vi "Read Channels Enqueuers.vi"(8 "error in (no error)":errorcluster, 11 "Sequencer in":refnum<class "Sequencer.lvclass">) -> (0 "error out":errorcluster, 2 "Channels Enqueuers":refnum<class "Message Enqueuer.lvclass">[](array[class]), 3 "Sequencer out":refnum<class "Sequencer.lvclass">)   [LabVIEW 2015, in "Sequencer.lvlib" / "Sequencer.lvclass"]
uses:
  Sequencer.lvclass
  <vilib>/ActorFramework/Message Enqueuer/Message Enqueuer.lvclass
  Sequencer.lvclass/Sequencer.ctl
  SequencerConfig.lvclass
  SequencerInfo.lvclass
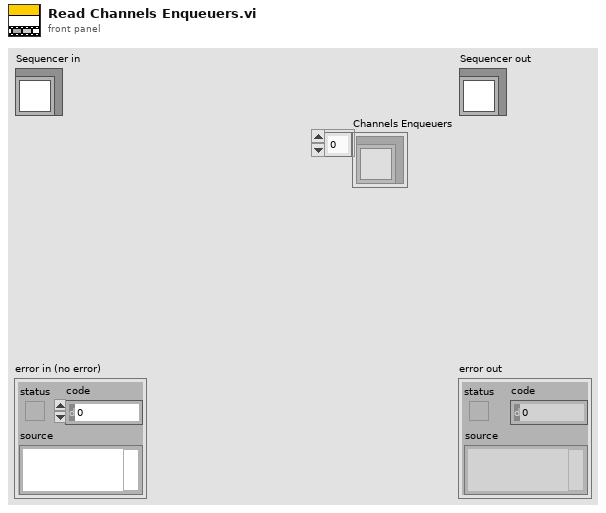
[diagram p1: front panel]
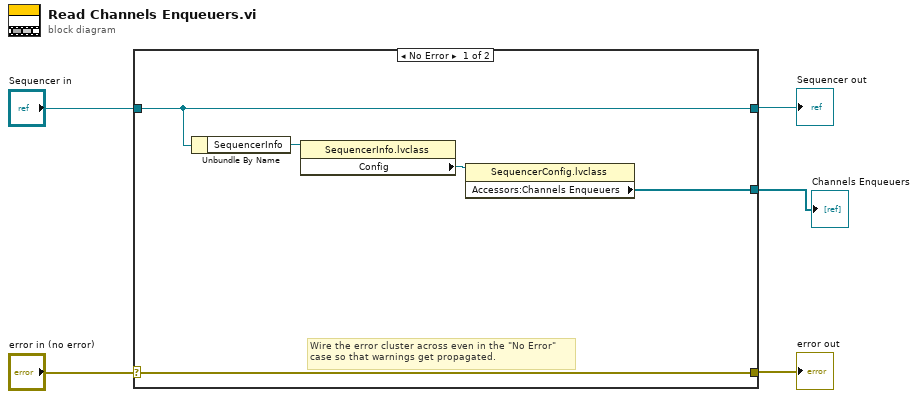
[diagram p0: block diagram]
diagram:
  n1 = case shown="No Error" "error in (no error)" {
    selector: "error in (no error)" -> [w10 w12]
    tunnel: [w10 w12] -> w4
    tunnel: [w8 w11] -> w2
    tunnel: "Sequencer in" -> [w8 w11]
    tunnel: [w6 _] -> w1
    frame No Error {
      # "Wire the error cluster across even in the \"No Error\"\ncase so that warnings get propagated."
      n2 = Unbundle By Name(w8) -> ("SequencerInfo"=w9:refnum<class "SequencerInfo.lvclass">)
      n3 = property class="SequencerInfo.lvclass"(reference=w9) -> ("Config"=w7:refnum<class "SequencerConfig.lvclass">)  [unwired: 1 in, 2 out]
      n4 = property class="SequencerConfig.lvclass"(reference=w7) -> ("Accessors:Channels Enqueuers"=w6:refnum<class "Message Enqueuer.lvclass">[])  [unwired: 1 in, 2 out]
    }
    frame Error {
    }
  }
  "error out" <- w4
  "Sequencer out" <- w2
  "Channels Enqueuers" <- w1
